vi "Borrow.vi"(8 "error in (no error)":errorcluster, 10 "Amount":dbl, 11 "ACreditAccount in":refnum<class "ACreditAccount.lvclass">) -> (0 "error out":errorcluster, 1 "Success?":bool, 2 "Balance":dbl, 3 "ACreditAccount out":refnum<class "ACreditAccount.lvclass">)   [LabVIEW 2020, in "ACreditAccount.lvclass"]
uses:
  ACreditAccount.lvclass
  ACreditAccount.lvclass/ACreditAccount.ctl
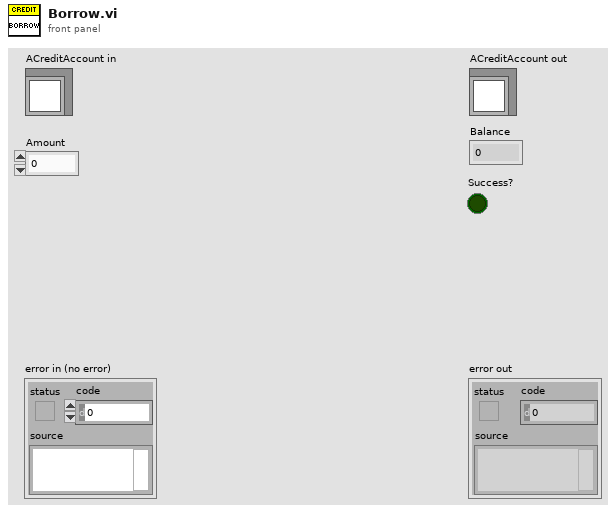
[diagram p1: front panel]
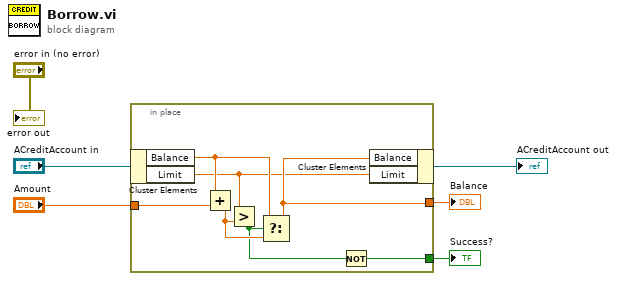
[diagram p0: block diagram]
diagram:
  n1 = in-place {
    in-place-border: "Amount" -> [w13]
    in-place-border: [w11] -> w3
    in-place-border: [w7] -> w2
    n2 = in-place-cluster #1("ACreditAccount in") -> ("Balance"=w12:dbl, "Limit"=w9:dbl)
    n3 = Add(x=w12, y=w13) -> (x+y=w10:dbl)
    n4 = Greater?(x=w9, y=w10) -> (0:w8:bool)
    n5 = Select(t=w12, s=w8, f=w10) -> (s? t:f=w11:dbl)
    n6 = Not(x=w8) -> (.not. x?=w7:bool)
    n7 = in-place-cluster #1("Balance"=w11, "Limit"=w9) -> (→"ACreditAccount out":refnum<class "ACreditAccount.lvclass">)
  }
  "Success?" <- w2
  "Balance" <- w3
  "error out" <- "error in (no error)"
